vi "Tank Filling.vi"() -> ()   [LabVIEW 2021]
panel:
  out "Slide 3":u8(slide) scale=0.0..100.0
  out "Slide 2":u8(slide) scale=0.0..100.0
  out "Slide":u8(slide) scale=0.0..100.0
  out "Tank 2":dbl(slide) scale=0.0..10.0
  out "Tank":dbl(slide) scale=0.0..10.0
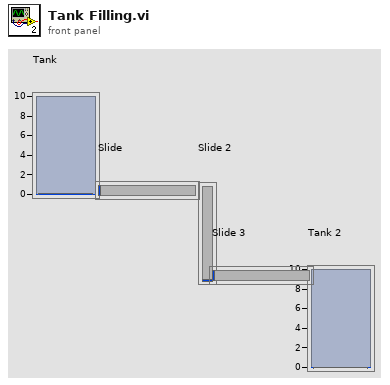
[diagram p1: front panel]
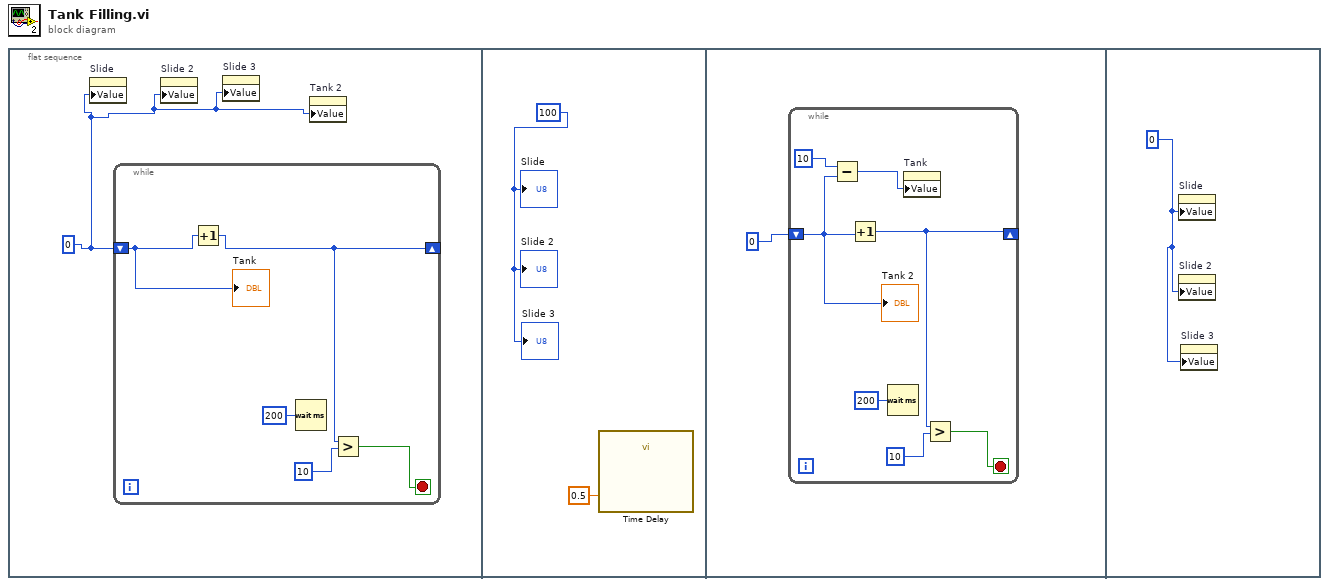
[diagram p0: block diagram]
diagram:
  n1 = flat-sequence {
    frame #0 {
      w1 = 0
      n2 = property on="Slide" class="Slide (strict)"("Value"=w1) -> ()  [unwired: 2 in, 2 out]
      n3 = while {
        shift-right: [w3] -> _
        shift-left: w1 -> [w4]
        stop <- w2 stop-if-true
        n4 = Increment(x=w4) -> (x+1=w3:i32)
        n5 = Wait (ms)(milliseconds to wait=u32 200) -> ()  [unwired: 1 out]
        n6 = Greater?(x=w3, y=10) -> (0:w2:bool)
        "Tank" <- w4
      }
      n7 = property on="Slide 2" class="Slide (strict)"("Value"=w1) -> ()  [unwired: 2 in, 2 out]
      n8 = property on="Slide 3" class="Slide (strict)"("Value"=w1) -> ()  [unwired: 2 in, 2 out]
      n9 = property on="Tank 2" class="Slide (strict)"("Value"=w1) -> ()  [unwired: 2 in, 2 out]
    }
    frame #1 {
      w8 = 100
      n10 = call "Time Delay"("Delay Time (s)"=0.5) -> ()  [unwired: 10 in, 1 out]
      "Slide" <- w8
      "Slide 2" <- w8
      "Slide 3" <- w8
    }
    frame #2 {
      n11 = while {
        shift-right: [w11] -> _
        shift-left: 0 -> [w15]
        stop <- w12 stop-if-true
        n12 = Subtract(x=10, y=w15) -> (x-y=w10:i32)
        n13 = Increment(x=w15) -> (x+1=w11:i32)
        n14 = Wait (ms)(milliseconds to wait=u32 200) -> ()  [unwired: 1 out]
        n15 = property on="Tank" class="Slide (strict)"("Value"=w10) -> ()  [unwired: 2 in, 2 out]
        n16 = Greater?(x=w11, y=10) -> (0:w12:bool)
        "Tank 2" <- w15
      }
    }
    frame #3 {
      w17 = 0
      n17 = property on="Slide" class="Slide (strict)"("Value"=w17) -> ()  [unwired: 2 in, 2 out]
      n18 = property on="Slide 2" class="Slide (strict)"("Value"=w17) -> ()  [unwired: 2 in, 2 out]
      n19 = property on="Slide 3" class="Slide (strict)"("Value"=w17) -> ()  [unwired: 2 in, 2 out]
    }
  }
